vi "Sort Bundles.vi"(8 "Error In":errorcluster, 11 "Bundles":cluster{"Label.Text":string, refnum<vi>}[](array[cluster])) -> (0 "Error Out":errorcluster, 3 "Sorted Elements":refnum<vi>[](array[refnum]))   [LabVIEW 2017, in "Toolkit.lvlib"]
uses:
  Toolkit.lvlib
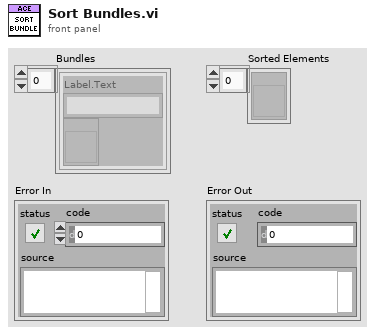
[diagram p1: front panel]
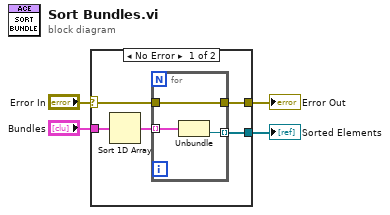
[diagram p0: block diagram]
diagram:
  n1 = case shown="No Error" "Error In" {
    selector: "Error In" -> [w5 w13]
    tunnel: "Bundles" -> [w9 _]
    tunnel: [w7 w13] -> w3
    tunnel: [w6 _] -> w2
    frame No Error {
      n2 = Sort 1D Array(array=w9) -> (sorted array=w8:cluster{"Label.Text":string, refnum<vi>}[])
      n3 = for {
        tunnel: w8 -> [w12] mode=indexing
        tunnel: w5 -> [w10]
        tunnel: [w11] -> w6 mode=indexing
        tunnel: [w10] -> w7
        n4 = Unbundle(w12) -> (w11:refnum<vi>)  [unwired: 1 out]
      }
    }
    frame Error {
    }
  }
  "Error Out" <- w3
  "Sorted Elements" <- w2
